vi "FilterAndSortData.vi"() -> ()   [LabVIEW 2018]
uses:
  <vilib>/Utility/file.llb/Read Delimited Spreadsheet (string).vi
panel:
  out "number":dbl[](array[numeric])
  in  "search string":string
  out "output array":string[][](array[string])
  out "parameter data":string[](array[string])
  out "filter data":string[](array[string])
  out "Parameter Index":i32
  in  "Parameter":string="RF_FREQ_OUT"
  in  "Filter":string="RF_FREQ_OUT"
  out "all rows":string[][](array[string])
  out "Filter index":i32
  out "Header":string[](array[string])
  out "Data":string[][](array[string])
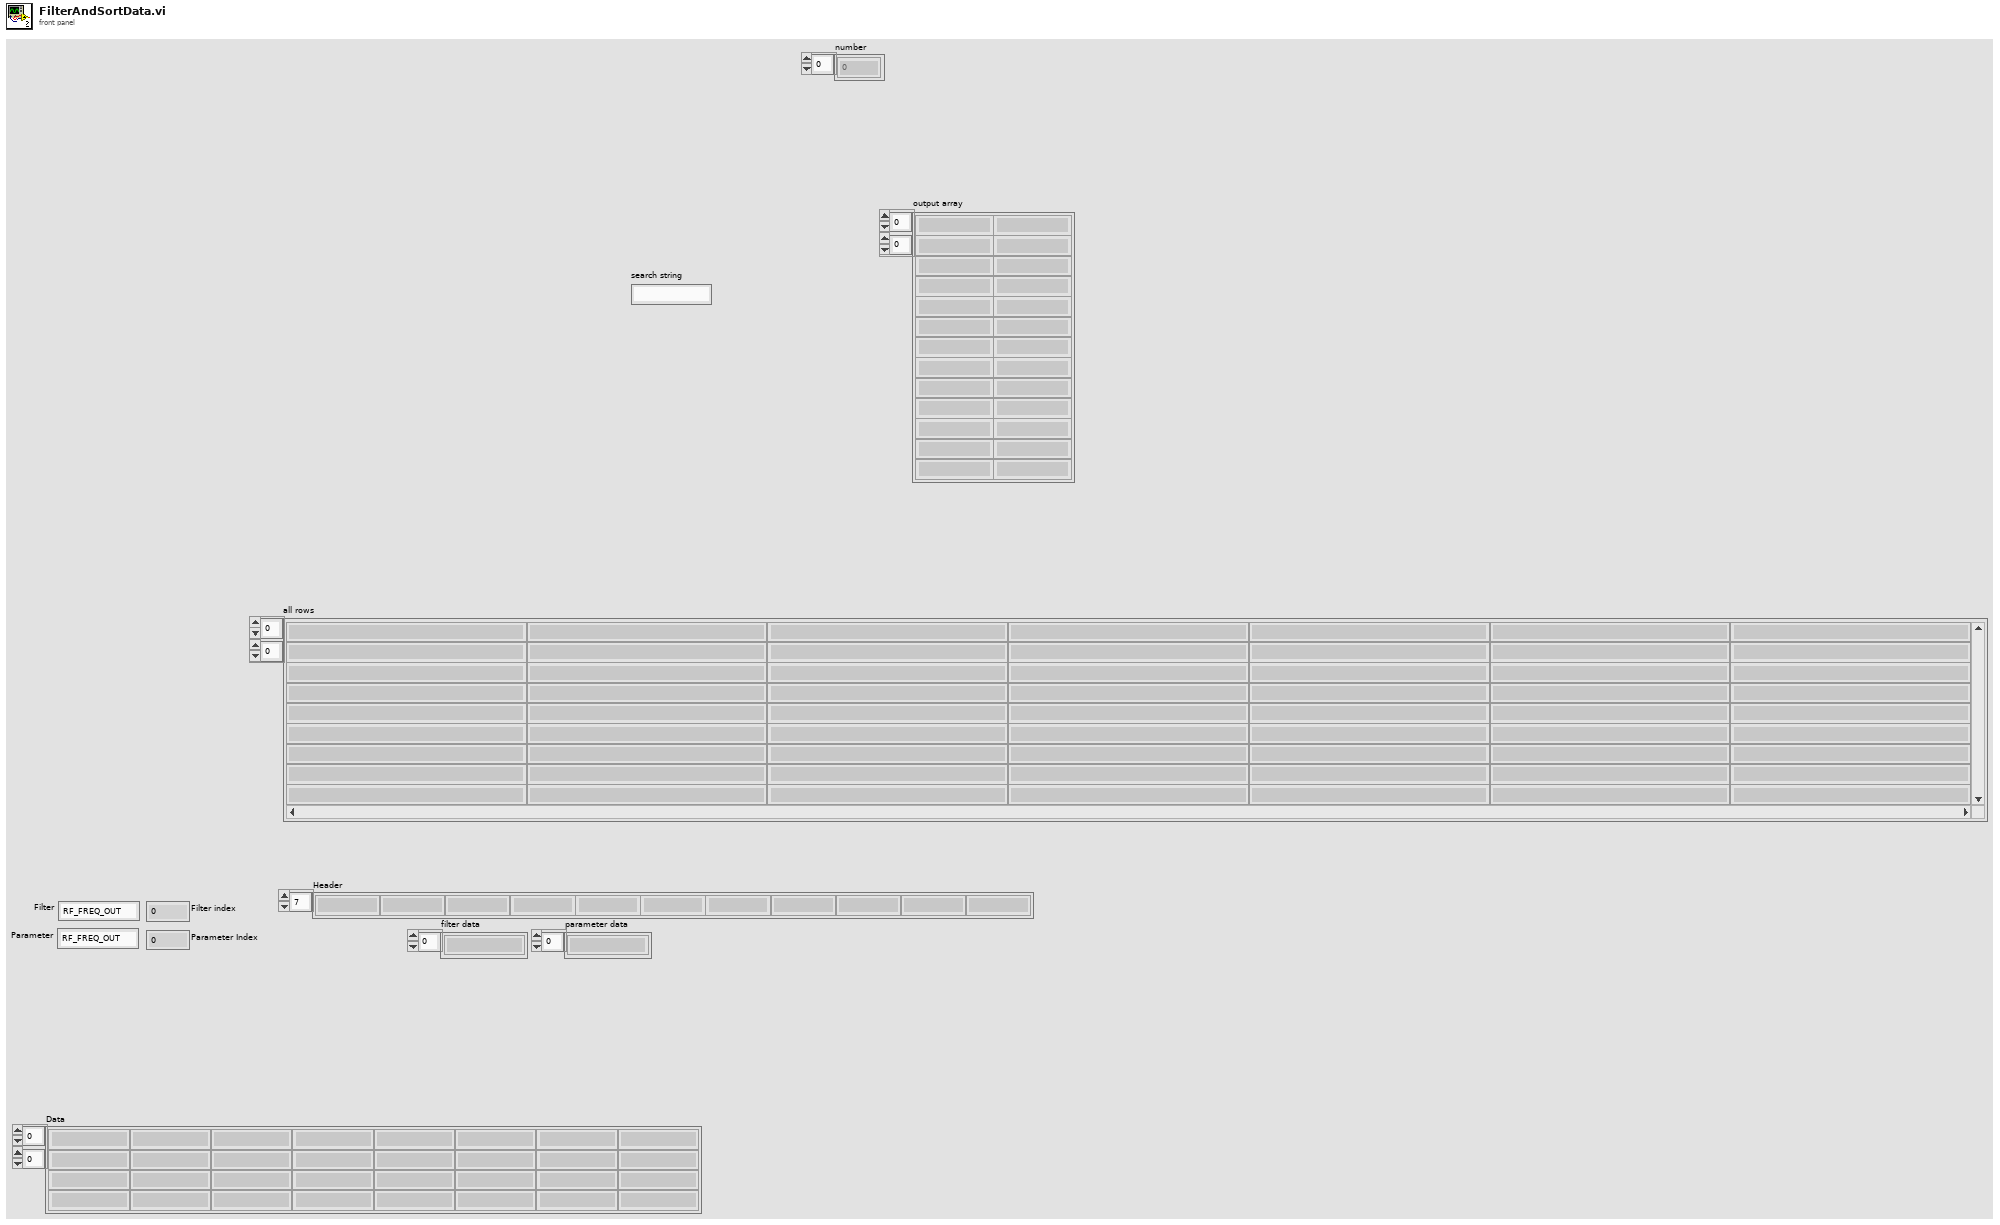
[diagram p1: front panel]
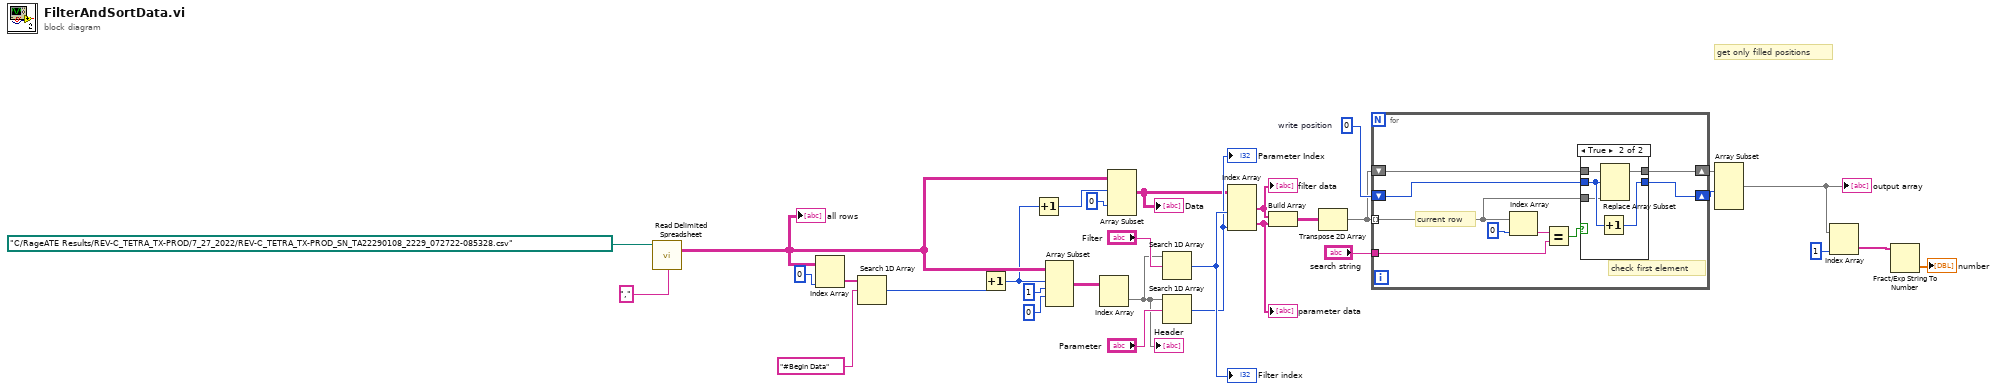
[diagram p0: block diagram]
diagram:
  w13 = 0  # write position
  # "get only filled positions"
  n1 = call-poly <vilib>:"Read Delimited Spreadsheet.vi"("file path (dialog if empty)"=path "C:/RageATE Results/REV-C_TETRA_TX-PROD/7_27_2022/REV-C_TETRA_TX-PROD_SN_TA22290108_2229_072722-085328.csv", "delimiter (\\t)"="," ("delimiter (\\t)")) -> ("all rows"=w23:string[][])  [unwired: 8 in, 5 out]
  "all rows" <- w23
  n2 = Index Array(array=w23, index (col)=0 ("disabled index (col)")) -> (element=w21:string[])  [unwired: 1 in]
  n3 = Search 1D Array(1D array=w21, element="#Begin Data") -> (index of element=w19:i32)  [unwired: 1 in]
  n4 = Increment(x=w19) -> (x+1=w18:i32)
  n5 = Increment(x=w18) -> (x+1=w24:i32)
  n6 = Array Subset(array=w23, index (row)=w18, length (row)=1 ("length"), index (col)=0 ("index")) -> (w26:string[][])  [unwired: 1 in]
  n7 = Index Array(array=w26) -> (element=w14:string[])  [unwired: 2 in]
  "Header" <- w14
  n8 = Array Subset(array=w23, index (row)=w24, index (col)=0 ("index")) -> (w7:string[][])  [unwired: 2 in]
  "Data" <- w7
  n9 = Search 1D Array(1D array=w14, element="Filter") -> (index of element=w17:i32)  [unwired: 1 in]
  "Filter index" <- w17
  n10 = Search 1D Array(1D array=w14, element="Parameter") -> (index of element=w15:i32)  [unwired: 1 in]
  "Parameter Index" <- w15
  n11 = Index Array(array=w7, index (col) #1=w17, index (col) #2=w15) -> (element #1=w9:string[], element #2=w8:string[])  [unwired: 2 in]
  "filter data" <- w9
  "parameter data" <- w8
  n12 = Build Array(w9, w8) -> (w6:string[][])
  n13 = Transpose 2D Array(2D array=w6) -> (transposed array=w5:string[][])
  n14 = for {
    shift-right: [w40] -> w11
    shift-left: w5 -> [w37]
    shift-right: [w38] -> w10
    shift-left: w13 -> [w39]
    tunnel: "search string" -> [w34]
    tunnel: w5 -> [w32] mode=indexing
    # "check first element"
    # "current row"
    n15 = Index Array(array=w32, index=0) -> (element=w35:string)
    n16 = Equal?(x=w35, y=w34) -> (x = y?=w33:bool)
    n17 = case shown="True" w33 {
      tunnel: w37 -> [w42 w47]
      tunnel: [w42 w46] -> w40
      tunnel: w39 -> [w41 w45]
      tunnel: [w41 w44] -> w38
      tunnel: w32 -> [_ w43]
      frame False {
      }
      frame True {
        n18 = Increment(x=w45) -> (x+1=w44:i32)
        n19 = Replace Array Subset(array=w47, new element=w43, index (row)=w45) -> (w46:string[][])  [unwired: 1 in]
      }
    }
  }
  n20 = Array Subset(array=w11, length (row)=w10) -> (w4:string[][])  [unwired: 3 in]
  "output array" <- w4
  n21 = Index Array(array=w4, index (col)=1 ("disabled index (col)")) -> (element=w2:string[])  [unwired: 1 in]
  n22 = Fract/Exp String To Number(string=w2) -> (number=→"number":dbl[])  [unwired: 3 in, 1 out]
